vi "Initialise.vi"(7 "Logger Name (Logger)":string="Logger", 11 "Handles":T1(c390)) -> ()   [LabVIEW 2024, in "RQMHLogSingleton.lvlib"]
uses:
  RQMHLogSingleton.lvlib
  RQMHLogger/RQMHLogger.lvclass
  LogHandle/Interface/LoggingHandle.lvclass
  HandleHolder/HandleHolder.lvclass
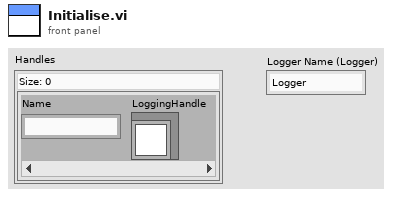
[diagram p1: front panel]
types:
  T1 = map{string, refnum<class "LoggingHandle.lvclass">}
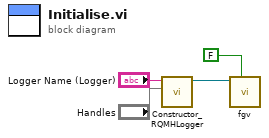
[diagram p0: block diagram]
diagram:
  n1 = call "Constructor_RQMHLogger.vi"("Handles"="Handles", "Name"="Logger Name (Logger)") -> ("RQMHLogger out"=w3:refnum<class "RQMHLogger.lvclass">)  [unwired: 8 in, 1 out]
  n2 = call "fgv.vi"("Get? (T)"=FALSE, "RQMHLogger Set"=w3) -> ()  [unwired: 9 in, 1 out]
